vi "ge trail1.vi"() -> ()   [LabVIEW 2014]
uses:
  <vilib>/LabVIEW Targets/FPGA/cRIO/shared/nicrio_ModuleControls/nicrio_cRIO-9225_DataRatesRing.ctl
  <vilib>/rvi/FXPMathLib/FxpSinAndCos/subVIs/nifxpmath_SinAndCos_SimConfig.ctl
  <vilib>/rvi/FXPMathLib/FxpRectToPolar/subVIs/nifxpmath_RectToPolar_SimConfig.ctl
  <vilib>/rvi/Emulation/niFpgaGetClockAttributes.vi
  <vilib>/rvi/Emulation/niFpgaSctlEmulationGetInTimedLoop.vi
  <vilib>/rvi/Emulation/niFpgaEmulationReportErrorSimple.vi
  <vilib>/rvi/eio/common/nirviEmuTemplateMethod_errors.vi
  <vilib>/rvi/Memory/Memory_Emulation/nirvimemoryFastEmulation.vi
  <vilib>/rvi/Memory/Memory_Emulation/nirvimemoryEmulation.vi
  <vilib>/rvi/Emulation/niFpgaEmulationIsFPGAContextNoSignature.vi
  <vilib>/rvi/DataTransferAndStorage/Container/Common/niFpgaContainerGetUniqueNameForEmu.vi
  <vilib>/rvi/Emulation/niFpgaProcessEmulError.vi
  <vilib>/rvi/errors/nirviReportUnexpectedCaseInternalError (U32).vi
  <vilib>/rvi/FXPMathLib/FxpSinAndCos/simVIs/DllFxpSinAndCosTemp_sub.vi
  <vilib>/rvi/FXPMathLib/FxpRectToPolar/simVIs/DllFxpRectToPolarTemp_sub.vi
  <vilib>/rvi/Emulation/niFpgaCriticalErrorInLSC.vi
  <vilib>/rvi/eio/common/nirviEmuTemplatePropertySet_noerrors.vi
  <vilib>/rvi/DataTransferAndStorage/Container/Common/niFpgaContainerSetEmuInfo.vi
  <vilib>/rvi/eio/common/nirviEmuReportErrorAndStop.vi
  <vilib>/eio/EIONode/EIONode.xnode
  <vilib>/rvi/DataTransferAndStorage/Container/XNode/niFpgaContainer.xnode
  <vilib>/rvi/FXPMathLib/FxpSub/XNode/nifxpmath_Sub.xnode
  <vilib>/rvi/FXPMathLib/FxpMul/XNode/nifxpmath_Multiplier.xnode
  <vilib>/rvi/FXPMathLib/FxpSinAndCos/XNode/nifxpmath_SinAndCos.xnode
  <vilib>/rvi/FXPMathLib/FxpAdd/XNode/nifxpmath_Add.xnode
  <vilib>/rvi/FXPMathLib/FxpRectToPolar/XNode/nifxpmath_RectToPolar.xnode
  <vilib>/eio/EIOPropertyNode/EIOPropertyNode.xnode
  <vilib>/LabVIEW Targets/FPGA/cRIO/shared/nicrio_ModuleControls/nicrio_cRIO-9227_DataRatesRing.ctl
  <vilib>/rvi/LocalResourceManager/LocalResourceManager.xnode
  <vilib>/rvi/eio/common/nirviEmuTemplatePropertyGet_errors.vi
  <vilib>/rvi/eio/common/nirviEmuTemplatePropertyGet_noerrors.vi
  <vilib>/rvi/eio/common/nirviEmuTemplatePropertySet_errors.vi
  <vilib>/rvi/FXPMathLib/sim/FxpSim.dll
panel:
  out "power factor":fxp<+/-,16,2>
  out "original power factor":fxp<+/-,16,2>
  out "current phase diff":fxp<+/-,26,12>
  out "voltage phase diff":fxp<+/-,26,12>
  out "final phase angle":fxp<+/-,16,2>[](array[numeric])
  out "final magnitude":fxp<+,30,12>[](array[numeric])
  out "imaginary value":fxp<+/-,59,16>[](array[numeric])
  out "real value":fxp<+/-,60,17>[](array[numeric])
  out "phase angle":fxp<+/-,22,10>[](array[numeric])
  out "magnitude":fxp<+,60,17>[](array[numeric])
  in  "stop":bool
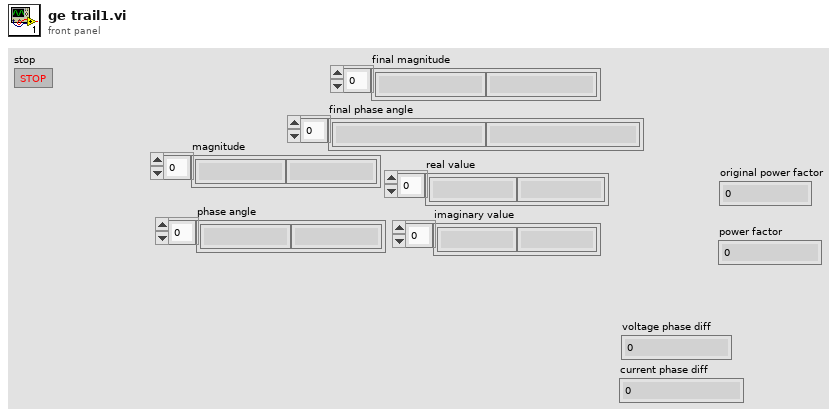
[diagram p1: front panel]
types:
  T1 = typedef "nicrio_cRIO-9225_DataRatesRing.ctl" = u8
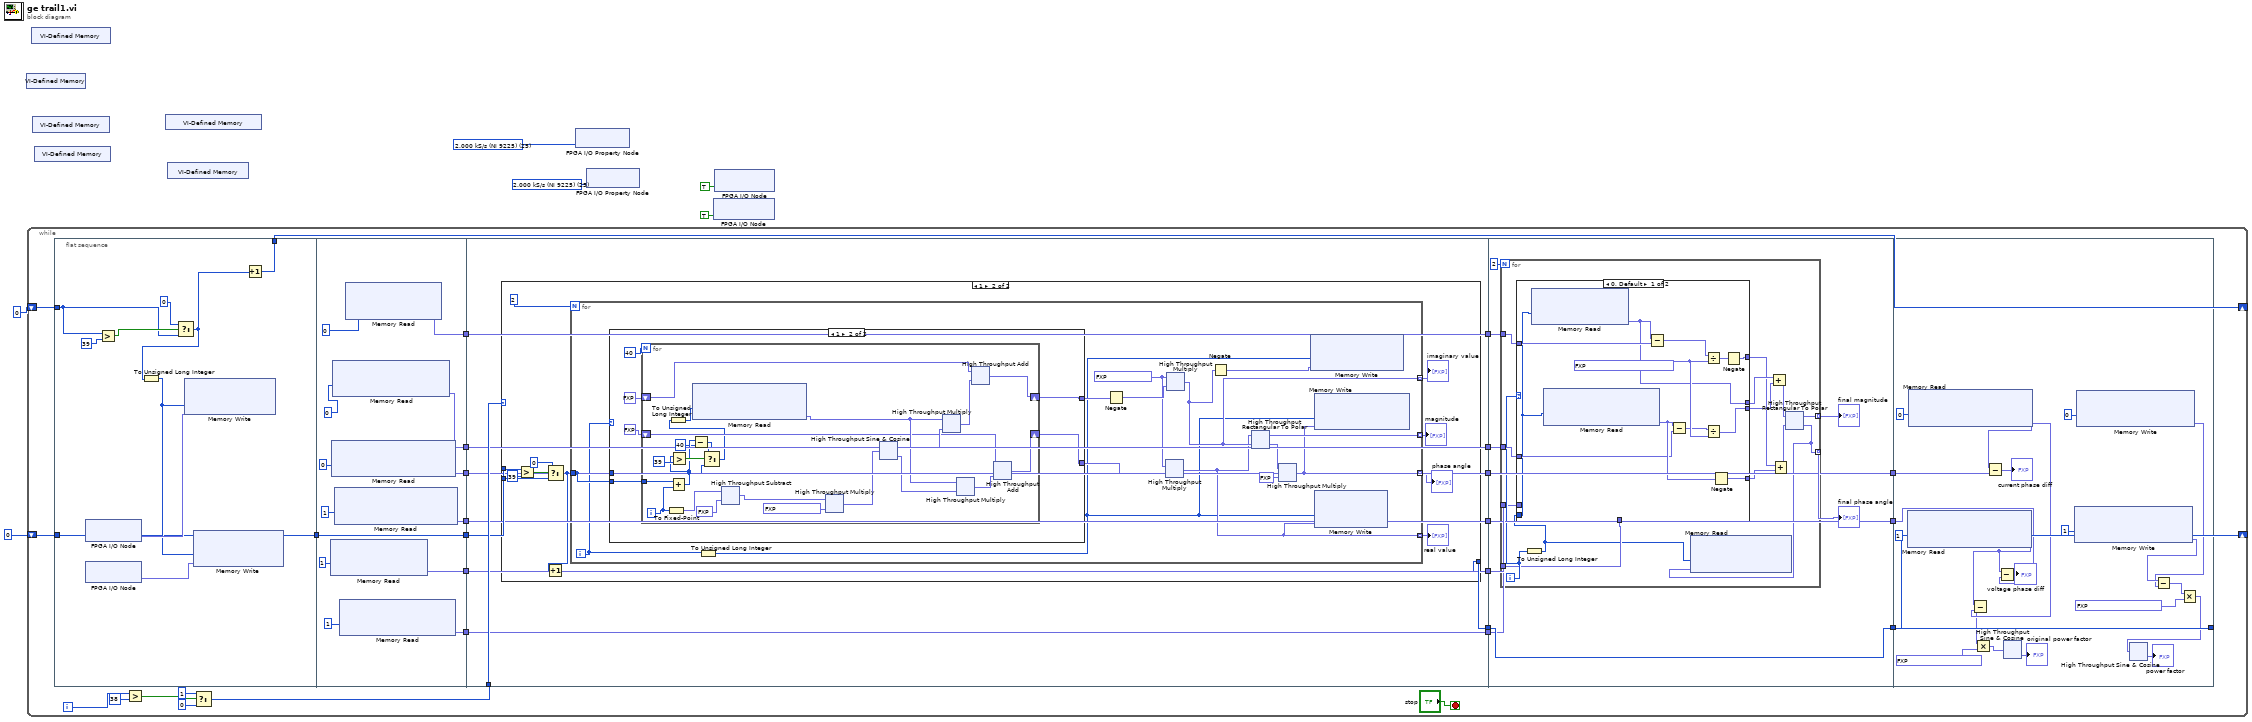
[diagram p0: block diagram]
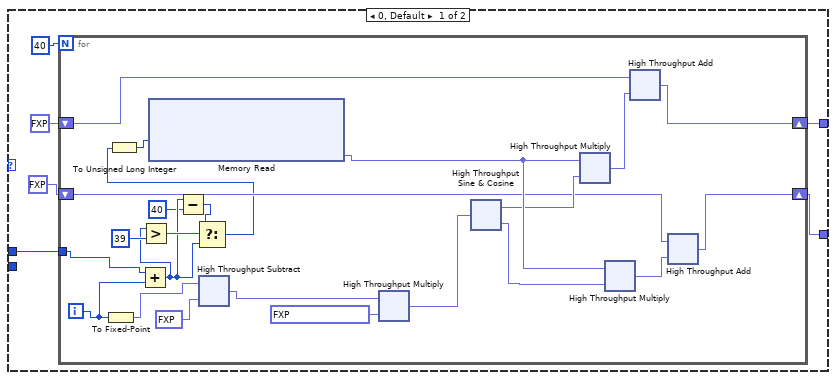
[diagram p3: hidden frame]
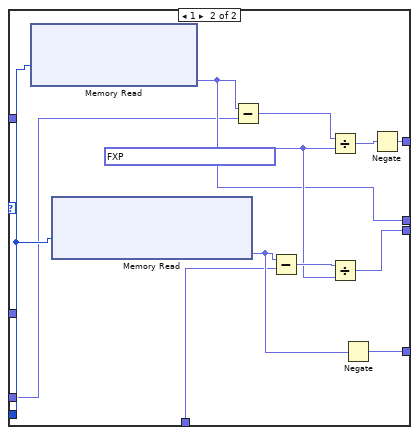
[diagram p4: hidden frame]
diagram:
  w3 = T1 25 items=["50.000 kS/s (NI 9225)"=1, "25.000 kS/s (NI 9225)"=2, "16.667 kS/s (NI 9225)"=3, "12.500 kS/s (NI 9225)"=4, "10.000 kS/s (NI 9225)"=5, "8.333 kS/s (NI 9225)"=6, "7.143 kS/s (NI 9225)"=7, "6.250 kS/s (NI 9225)"=8, "5.556 kS/s (NI 9225)"=9, "5.000 kS/s (NI 9225)"=10, "4.545 kS/s (NI 9225)"=11, "4.167 kS/s (NI 9225)"=12, "3.846 kS/s (NI 9225)"=13, "3.571 kS/s (NI 9225)"=14, "3.333 kS/s (NI 9225)"=15, "3.125 kS/s (NI 9225)"=16, "2.941 kS/s (NI 9225)"=17, "2.778 kS/s (NI 9225)"=18, "2.632 kS/s (NI 9225)"=19, "2.500 kS/s (NI 9225)"=20, "2.381 kS/s (NI 9225)"=21, "2.273 kS/s (NI 9225)"=22, "2.174 kS/s (NI 9225)"=23, "2.083 kS/s (NI 9225)"=24, "2.000 kS/s (NI 9225)"=25, "1.923 kS/s (NI 9225)"=26, "1.852 kS/s (NI 9225)"=27, "1.786 kS/s (NI 9225)"=28, "1.724 kS/s (NI 9225)"=29, "1.667 kS/s (NI 9225)"=30, "1.613 kS/s (NI 9225)"=31] ("Data Rate")
  w4 = T1 25 items=["50.000 kS/s (NI 9225)"=1, "25.000 kS/s (NI 9225)"=2, "16.667 kS/s (NI 9225)"=3, "12.500 kS/s (NI 9225)"=4, "10.000 kS/s (NI 9225)"=5, "8.333 kS/s (NI 9225)"=6, "7.143 kS/s (NI 9225)"=7, "6.250 kS/s (NI 9225)"=8, "5.556 kS/s (NI 9225)"=9, "5.000 kS/s (NI 9225)"=10, "4.545 kS/s (NI 9225)"=11, "4.167 kS/s (NI 9225)"=12, "3.846 kS/s (NI 9225)"=13, "3.571 kS/s (NI 9225)"=14, "3.333 kS/s (NI 9225)"=15, "3.125 kS/s (NI 9225)"=16, "2.941 kS/s (NI 9225)"=17, "2.778 kS/s (NI 9225)"=18, "2.632 kS/s (NI 9225)"=19, "2.500 kS/s (NI 9225)"=20, "2.381 kS/s (NI 9225)"=21, "2.273 kS/s (NI 9225)"=22, "2.174 kS/s (NI 9225)"=23, "2.083 kS/s (NI 9225)"=24, "2.000 kS/s (NI 9225)"=25, "1.923 kS/s (NI 9225)"=26, "1.852 kS/s (NI 9225)"=27, "1.786 kS/s (NI 9225)"=28, "1.724 kS/s (NI 9225)"=29, "1.667 kS/s (NI 9225)"=30, "1.613 kS/s (NI 9225)"=31] ("Data Rate")
  n1 = xnode "VI-Defined Memory"() -> ()  [unwired: 1 out]
  n2 = while {
    shift-right: [w34] -> _
    shift-left: i16 0 -> [w33]
    shift-right: [w25] -> _
    shift-left: u32 0 -> [w26]
    i -> [w32]
    stop <- "stop" stop-if-true
    n3 = flat-sequence {
      tunnel: [w43] -> w34
      tunnel: w33 -> [w39]
      tunnel: [w36] -> w24
      tunnel: w26 -> [w36]
      tunnel: w24 -> [w58]
      tunnel: [w58] -> w23
      tunnel: [w55] -> w21
      tunnel: [w54] -> w18
      tunnel: [w51] -> w16
      tunnel: [w50] -> w14
      tunnel: [w47] -> w12
      tunnel: [w46] -> w7
      tunnel: w27 -> [w67]
      tunnel: w23 -> [w65]
      tunnel: [w66] -> w22
      tunnel: w21 -> [w64]
      tunnel: [w64] -> w20
      tunnel: [w63] -> w19
      tunnel: w18 -> [w63]
      tunnel: [w62] -> w17
      tunnel: w16 -> [w62]
      tunnel: [w59] -> w15
      tunnel: w14 -> [w59]
      tunnel: w12 -> [w61]
      tunnel: [w61] -> w11
      tunnel: [w60] -> w8
      tunnel: w7 -> [w60]
      tunnel: w22 -> [w259]
      tunnel: w20 -> [w257]
      tunnel: w19 -> [w256]
      tunnel: w17 -> [w253]
      tunnel: w15 -> [w252]
      tunnel: [w259] -> w13
      tunnel: w11 -> [w251]
      tunnel: [w251] -> w10
      tunnel: [w250] -> w9
      tunnel: w8 -> [w250]
      tunnel: [w355] -> w25
      tunnel: w13 -> [w355]
      tunnel: w10 -> [w352]
      tunnel: w9 -> [w351]
      frame #0 {
        n4 = xnode "FPGA I/O Node"() -> ("Mod1/AI1"=w44:fxp<+/-,24,10>)  [unwired: 1 in, 1 out]
        n5 = xnode "FPGA I/O Node"() -> ("Mod2/AI1"=w45:fxp<+/-,24,5>)  [unwired: 1 in, 1 out]
        n6 = Greater?(x=w39, y=i16 39) -> (0:w41:bool)
        n7 = Select(t=i16 0, s=w41, f=w39) -> (s? t:f=w38:i16)
        n8 = To Unsigned Long Integer(number=w38) -> (unsigned 32bit integer=w37:u32)
        n9 = xnode ("Memory Write")("Address"=w37, "Data"=w44) -> ()  [unwired: 1 in, 1 out]
        n10 = xnode ("Memory Write")("Address"=w37, "Data"=w45) -> ()  [unwired: 1 in, 1 out]
        n11 = Increment(x=w38) -> (x+1=w43:i16)
      }
      frame #1 {
        n12 = xnode ("Memory Read")("Address"=u32 1) -> ("Data"=w51:fxp<+/-,25,11>)  [unwired: 1 in, 1 out]
        n13 = xnode ("Memory Read")("Address"=u32 0) -> ("Data"=w47:fxp<+/-,25,11>)  [unwired: 1 in, 1 out]
        n14 = xnode ("Memory Read")("Address"=u32 0) -> ("Data"=w54:fxp<+/-,25,11>)  [unwired: 1 in, 1 out]
        n15 = xnode ("Memory Read")("Address"=u32 1) -> ("Data"=w46:fxp<+/-,25,11>)  [unwired: 1 in, 1 out]
        n16 = xnode ("Memory Read")("Address"=u32 1) -> ("Data"=w50:fxp<+/-,25,11>)  [unwired: 1 in, 1 out]
        n17 = xnode ("Memory Read")("Address"=u32 0) -> ("Data"=w55:fxp<+/-,25,11>)  [unwired: 1 in, 1 out]
      }
      frame #2 {
        n18 = case shown="1" w67 {
          tunnel: w65 -> [w68 w74]
          tunnel: [w68 w75] -> w66
          tunnel: w65 -> [_ w70]
          frame 0, Default {
          }
          frame 1 {
            n19 = Greater?(x=w74, y=u32 39) -> (0:w72:bool)
            n20 = Select(t=u32 0, s=w72, f=w70) -> (s? t:f=w69:u32)
            n21 = Increment(x=w69) -> (x+1=w75:u32)
            n22 = for {
              N: 2 -> [_]
              tunnel: [w89] -> w79 mode=indexing
              tunnel: [w81] -> w78 mode=indexing
              tunnel: [w84] -> w77 mode=indexing
              tunnel: [w86] -> w76 mode=indexing
              tunnel: w69 -> [w88]
              i -> [w87]
              w83 = fxp<+/-,16,1> 0.03533935546875 ("x")
              n23 = case shown="1" w87 {
                tunnel: [w134 w193] -> w94
                tunnel: [w133 w192] -> w92
                tunnel: w88 -> [w132 _]
                tunnel: w88 -> [_ w191]
                frame 0, Default {
                  n24 = for {
                    N: 40 -> [_]
                    shift-right: [w151] -> w134
                    shift-left: fxp<+/-,42,14> 0.0 ("x+y") -> [w150]
                    shift-right: [w149] -> w133
                    shift-left: fxp<+/-,44,16> 0.0 ("x+y") -> [w148]
                    tunnel: w132 -> [w141]
                    i -> [w142]
                    n25 = To Fixed-Point(number=w142) -> (fixed-point=w159:fxp<+/-,32,32>)  [unwired: 1 in]
                    n26 = Add(x=w141, y=w142) -> (x+y=w145:u32)
                    n27 = Greater?(x=w145, y=u32 39) -> (0:w146:bool)
                    n28 = Subtract(x=w145, y=u32 40) -> (x-y=w143:u32)
                    n29 = Select(t=w143, s=w146, f=w145) -> (s? t:f=w139:u32)
                    n30 = To Unsigned Long Integer(number=w139) -> (unsigned 32bit integer=w140:u32)
                    n31 = xnode ("Memory Read")("Address"=w140) -> ("Data"=w153:fxp<+/-,25,11>)  [unwired: 1 in, 1 out]
                    n32 = xnode "High Throughput Subtract"("x"=w159, "y"=fxp<+,6,5> 19.5) -> ("x-y"=w158:fxp<+/-,34,33>)
                    n33 = xnode ("High Throughput Multiply")("x"=w158, "y"=fxp<+,45,-4> 0.04998779296875) -> ("x*y"=w156:fxp<+/-,64,29>)
                    n34 = xnode "High Throughput Sine & Cosine"("x (pi)"=w156) -> ("sin(x)"=w152:fxp<+/-,16,2>, "cos(x)"=w138:fxp<+/-,16,2>)
                    n35 = xnode ("High Throughput Multiply")("x"=w153, "y"=w152) -> ("x*y"=w155:fxp<+/-,41,13>)
                    n36 = xnode ("High Throughput Multiply")("x"=w153, "y"=w138) -> ("x*y"=w154:fxp<+/-,41,13>)
                    n37 = xnode ("High Throughput Add")("x"=w150, "y"=w155) -> ("x+y"=w151:fxp<+/-,42,14>)
                    n38 = xnode ("High Throughput Add")("x"=w148, "y"=w154) -> ("x+y"=w149:fxp<+/-,44,16>)
                  }
                }
                frame 1 {
                  n39 = for {
                    N: 40 -> [_]
                    shift-right: [w210] -> w193
                    shift-left: fxp<+/-,42,14> 0.0 ("x+y") -> [w209]
                    shift-right: [w207] -> w192
                    shift-left: fxp<+/-,44,16> 0.0 ("x+y") -> [w208]
                    tunnel: w191 -> [w198]
                    i -> [w201]
                    n40 = To Fixed-Point(number=w201) -> (fixed-point=w212:fxp<+/-,32,32>)  [unwired: 1 in]
                    n41 = Add(x=w198, y=w201) -> (x+y=w204:u32)
                    n42 = Greater?(x=w204, y=u32 39) -> (0:w205:bool)
                    n43 = Subtract(x=w204, y=u32 40) -> (x-y=w202:u32)
                    n44 = Select(t=w202, s=w205, f=w204) -> (s? t:f=w199:u32)
                    n45 = To Unsigned Long Integer(number=w199) -> (unsigned 32bit integer=w200:u32)
                    n46 = xnode ("Memory Read")("Address"=w200) -> ("Data"=w218:fxp<+/-,25,11>)  [unwired: 1 in, 1 out]
                    n47 = xnode "High Throughput Subtract"("x"=w212, "y"=fxp<+,6,5> 19.5) -> ("x-y"=w213:fxp<+/-,34,33>)
                    n48 = xnode ("High Throughput Multiply")("x"=w213, "y"=fxp<+,45,-4> 0.04998779296875) -> ("x*y"=w215:fxp<+/-,64,29>)
                    n49 = xnode "High Throughput Sine & Cosine"("x (pi)"=w215) -> ("sin(x)"=w219:fxp<+/-,16,2>, "cos(x)"=w197:fxp<+/-,16,2>)
                    n50 = xnode ("High Throughput Multiply")("x"=w218, "y"=w219) -> ("x*y"=w216:fxp<+/-,41,13>)
                    n51 = xnode ("High Throughput Multiply")("x"=w218, "y"=w197) -> ("x*y"=w217:fxp<+/-,41,13>)
                    n52 = xnode ("High Throughput Add")("x"=w209, "y"=w216) -> ("x+y"=w210:fxp<+/-,42,14>)
                    n53 = xnode ("High Throughput Add")("x"=w208, "y"=w217) -> ("x+y"=w207:fxp<+/-,44,16>)
                  }
                }
              }
              n54 = To Unsigned Long Integer(number=w87) -> (unsigned 32bit integer=w82:u32)
              n55 = Negate(x=w94) -> (-x=w93:fxp<+/-,43,15>)
              n56 = xnode ("High Throughput Multiply")("x"=w83, "y"=w92) -> ("x*y"=w84:fxp<+/-,60,17>)
              n57 = xnode ("High Throughput Multiply")("x"=w83, "y"=w93) -> ("x*y"=w86:fxp<+/-,59,16>)
              n58 = Negate(x=w86) -> (-x=w85:fxp<+/-,60,17>)
              n59 = xnode "High Throughput Rectangular To Polar"("x"=w84, "y"=w86) -> ("magnitude"=w89:fxp<+,60,17>, "phase (pi)"=w91:fxp<+/-,16,2>)
              n60 = xnode ("High Throughput Multiply")("x"=w91, "y"=fxp<+,6,8> 180.0) -> ("x*y"=w81:fxp<+/-,22,10>)
              n61 = xnode ("Memory Write")("Address"=w82, "Data"=w85) -> ()  [unwired: 1 in, 1 out]
              n62 = xnode ("Memory Write")("Address"=w82, "Data"=w84) -> ()  [unwired: 1 in, 1 out]
              n63 = xnode ("Memory Write")("Address"=w82, "Data"=w81) -> ()  [unwired: 1 in, 1 out]
            }
            "magnitude" <- w79
            "phase angle" <- w78
            "real value" <- w77
            "imaginary value" <- w76
          }
        }
      }
      frame #3 {
        n64 = for {
          N: 2 -> [_]
          tunnel: w257 -> [w273]
          tunnel: w256 -> [w272]
          tunnel: [w265] -> w255 mode=indexing
          tunnel: [w260] -> w254 mode=indexing
          tunnel: w253 -> [w263]
          tunnel: w252 -> [w262]
          i -> [w264]
          n65 = To Unsigned Long Integer(number=w264) -> (unsigned 32bit integer=w261:u32)
          n66 = case shown="0, Default" w264 {
            tunnel: w261 -> [w278 w297]
            tunnel: w273 -> [w280 _]
            tunnel: w272 -> [w279 _]
            tunnel: [w276 w292] -> w271
            tunnel: [w277 w291] -> w270
            tunnel: [w274 w289] -> w269
            tunnel: [w275 w288] -> w268
            tunnel: w263 -> [_ w287]
            tunnel: w262 -> [_ w286]
            frame 0, Default {
              w283 = fxp<+,29,4> 12.514757186174393 ("y")
              n67 = xnode ("Memory Read")("Address"=w278) -> ("Data"=w277:fxp<+/-,25,11>)  [unwired: 1 in, 1 out]
              n68 = xnode ("Memory Read")("Address"=w278) -> ("Data"=w284:fxp<+/-,25,11>)  [unwired: 1 in, 1 out]
              n69 = Subtract(x=w277, y=w280) -> (x-y=w281:fxp<+/-,26,12>)
              n70 = Subtract(x=w284, y=w279) -> (x-y=w282:fxp<+/-,26,12>)
              n71 = Divide(x=w281, y=w283) -> (x/y=w285:fxp<+/-,27,9>)
              n72 = Divide(x=w282, y=w283) -> (x/y=w276:fxp<+/-,27,9>)
              n73 = Negate(x=w284) -> (-x=w275:fxp<+/-,26,12>)
              n74 = Negate(x=w285) -> (-x=w274:fxp<+/-,27,9>)
            }
            frame 1 {
              w294 = fxp<+,29,4> 12.514757186174393 ("y")
              n75 = xnode ("Memory Read")("Address"=w297) -> ("Data"=w291:fxp<+/-,25,11>)  [unwired: 1 in, 1 out]
              n76 = xnode ("Memory Read")("Address"=w297) -> ("Data"=w293:fxp<+/-,25,11>)  [unwired: 1 in, 1 out]
              n77 = Subtract(x=w291, y=w287) -> (x-y=w296:fxp<+/-,26,12>)
              n78 = Subtract(x=w293, y=w286) -> (x-y=w295:fxp<+/-,26,12>)
              n79 = Divide(x=w296, y=w294) -> (x/y=w290:fxp<+/-,27,9>)
              n80 = Divide(x=w295, y=w294) -> (x/y=w292:fxp<+/-,27,9>)
              n81 = Negate(x=w293) -> (-x=w288:fxp<+/-,26,12>)
              n82 = Negate(x=w290) -> (-x=w289:fxp<+/-,27,9>)
            }
          }
          n83 = Add(x=w270, y=w271) -> (x+y=w266:fxp<+/-,30,12>)
          n84 = Add(x=w269, y=w268) -> (x+y=w267:fxp<+/-,30,12>)
          n85 = xnode "High Throughput Rectangular To Polar"("x"=w266, "y"=w267) -> ("magnitude"=w265:fxp<+,30,12>, "phase (pi)"=w260:fxp<+/-,16,2>)
          n86 = xnode ("Memory Read")("Address"=w261, "Data"=w260) -> ()  [unwired: 1 in, 1 out]
        }
        "final magnitude" <- w255
        "final phase angle" <- w254
      }
      frame #4 {
        n87 = xnode ("Memory Read")("Address"=u32 1) -> ("Data"=w348:fxp<+/-,25,11>)  [unwired: 1 in, 1 out]
        n88 = xnode ("Memory Read")("Address"=u32 0) -> ("Data"=w347:fxp<+/-,25,11>)  [unwired: 1 in, 1 out]
        n89 = Subtract(x=w348, y=w347) -> (x-y=w345:fxp<+/-,26,12>)
        n90 = Multiply(x=w345, y=fxp<+,15,-7> 0.005554914474487305) -> (x*y=w346:fxp<+/-,41,5>)
        n91 = Subtract(x=w347, y=w352) -> (x-y=→"current phase diff":fxp<+/-,26,12>)
        n92 = Subtract(x=w348, y=w351) -> (x-y=→"voltage phase diff":fxp<+/-,26,12>)
        n93 = xnode "High Throughput Sine & Cosine"("x (pi)"=w346) -> ("cos(x)"=→"original power factor":fxp<+/-,16,2>)  [unwired: 1 out]
        n94 = xnode ("Memory Write")("Address"=u32 1) -> ("Data"=w337:fxp<+/-,25,11>)  [unwired: 1 in, 1 out]
        n95 = xnode ("Memory Write")("Address"=u32 0) -> ("Data"=w336:fxp<+/-,25,11>)  [unwired: 1 in, 1 out]
        n96 = Subtract(x=w337, y=w336) -> (x-y=w338:fxp<+/-,26,12>)
        n97 = Multiply(x=w338, y=fxp<+,15,-7> 0.005554914474487305) -> (x*y=w335:fxp<+/-,41,5>)
        n98 = xnode "High Throughput Sine & Cosine"("x (pi)"=w335) -> ("cos(x)"=→"power factor":fxp<+/-,16,2>)  [unwired: 1 out]
      }
    }
    n99 = Greater?(x=w32, y=38) -> (0:w30:bool)
    n100 = Select(t=i16 1, s=w30, f=i16 0) -> (s? t:f=w27:i16)
  }
  n101 = xnode "VI-Defined Memory"() -> ()  [unwired: 1 out]
  n102 = xnode "VI-Defined Memory"() -> ()  [unwired: 1 out]
  n103 = xnode "VI-Defined Memory"() -> ()  [unwired: 1 out]
  n104 = xnode "VI-Defined Memory"() -> ()  [unwired: 1 out]
  n105 = xnode "VI-Defined Memory"() -> ()  [unwired: 1 out]
  n106 = xnode "FPGA I/O Property Node"("Data Rate"=w4) -> ()  [unwired: 1 in, 1 out]
  n107 = xnode "FPGA I/O Property Node"("Data Rate"=w3) -> ()  [unwired: 1 in, 1 out]
  n108 = xnode "FPGA I/O Node"("Mod2/Start"=TRUE) -> ()  [unwired: 1 in, 1 out]
  n109 = xnode "FPGA I/O Node"("Mod1/Start"=TRUE) -> ()  [unwired: 1 in, 1 out]
